vi "LWXPS_EventExtendedRemove.vi"(6 "LabVIEW error IN":errorcluster caption="LabVIEW error IN\nLabVIEW error IN\nLabVIEW error IN", 8 "ID":i32, 9 "XPS Reference IN":refnum<k24>) -> (0 "LabVIEW error OUT":errorcluster, 1 "XPS Error String":string, 2 "Returned error code":i32, 3 "XPS Reference OUT":refnum<k24>)   [LabVIEW 2014]
uses:
  D:/XPSQ8_LabView_Library/Development/Source/Dll/Newport.XPS.CommandInterface.dll
  Dll/Newport.XPS.CommandInterface.dll
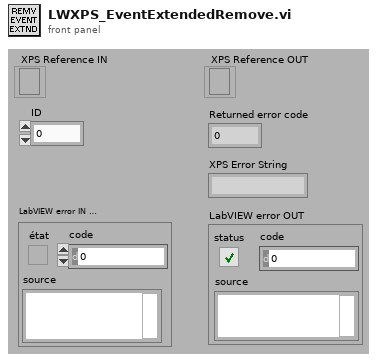
[diagram p1: front panel]
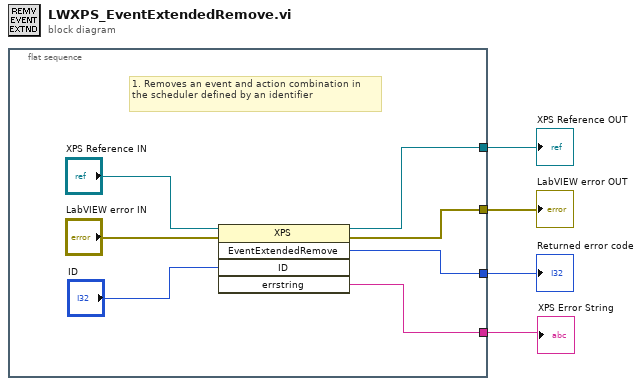
[diagram p0: block diagram]
diagram:
  n1 = flat-sequence {
    tunnel: [w10] -> w4
    tunnel: [w9] -> w3
    tunnel: [w6] -> w2
    tunnel: [w5] -> w1
    frame #0 {
      # "1. Removes an event and action combination in the scheduler defined by an identifier"
      n2 = invoke class="XPS" method="EventExtendedRemove"(reference="XPS Reference IN", error in="LabVIEW error IN", "ID"="ID") -> (reference out=w10:refnum<k24>, error out=w9:errorcluster, "EventExtendedRemove"=w5:i32, "errstring"=w6:string)  [unwired: 2 in, 1 out]
    }
  }
  "XPS Reference OUT" <- w4
  "LabVIEW error OUT" <- w3
  "XPS Error String" <- w2
  "Returned error code" <- w1
